vi "VI_Heat_Tape.vi"() -> ()   [LabVIEW 2019]
uses:
  <vilib>/NI/Modbus Library/API/Wrapper/Create Serial Master.vi
  <vilib>/NI/Modbus Library/API/Master/Modbus Master.lvclass
  <vilib>/NI/Modbus Library/API/Wrapper/API Main.lvlib
  <vilib>/NI/Modbus Library/Transmission Data Unit/RTU/RTU Data Unit.lvclass
panel:
  out "Alarm Status":bool
  out "Waveform Chart":dbl(graph)
  out "PXF4 Status":bool
  out "Heater Status":bool
  in  "Upper Threshold (ºF)":string
  in  "Lower Threshold (ºF)":string
  out "Current Temperature Status":bool
  in  "?":bool
  out "Current Temperature (ºF)":string
  out "Heat Tape Temperature (ºF)":dbl(slide) scale=70.0..80.0
  out "Value":sgl
  out "Response Message":string
  out "data string":string
  out "Query Message":string
  in  "unit ID":u8=1
  out "Register and RAW value":u16[](array[numeric])
  in  "number of inputs":u16
  in  "starting address":u16
  in  "error in":errorcluster
  in  "Flow Control":u16(ring) items=["None", "XON/XOFF", "RTS/CTS", "XON/XOFF & RTS/CTS", "DTR/DSR", "XON/XOFF & DTR/DSR"]
  in  "Serial Type":enum16{"RTU", "ASCII"}(ring)
  in  "Parity":u16(ring)=2 items=["None", "Odd", "Even", "Mark", "Space"]
  in  "Baud Rate":u32=9600
  in  "COM Port":refnum<visa-resource-name>
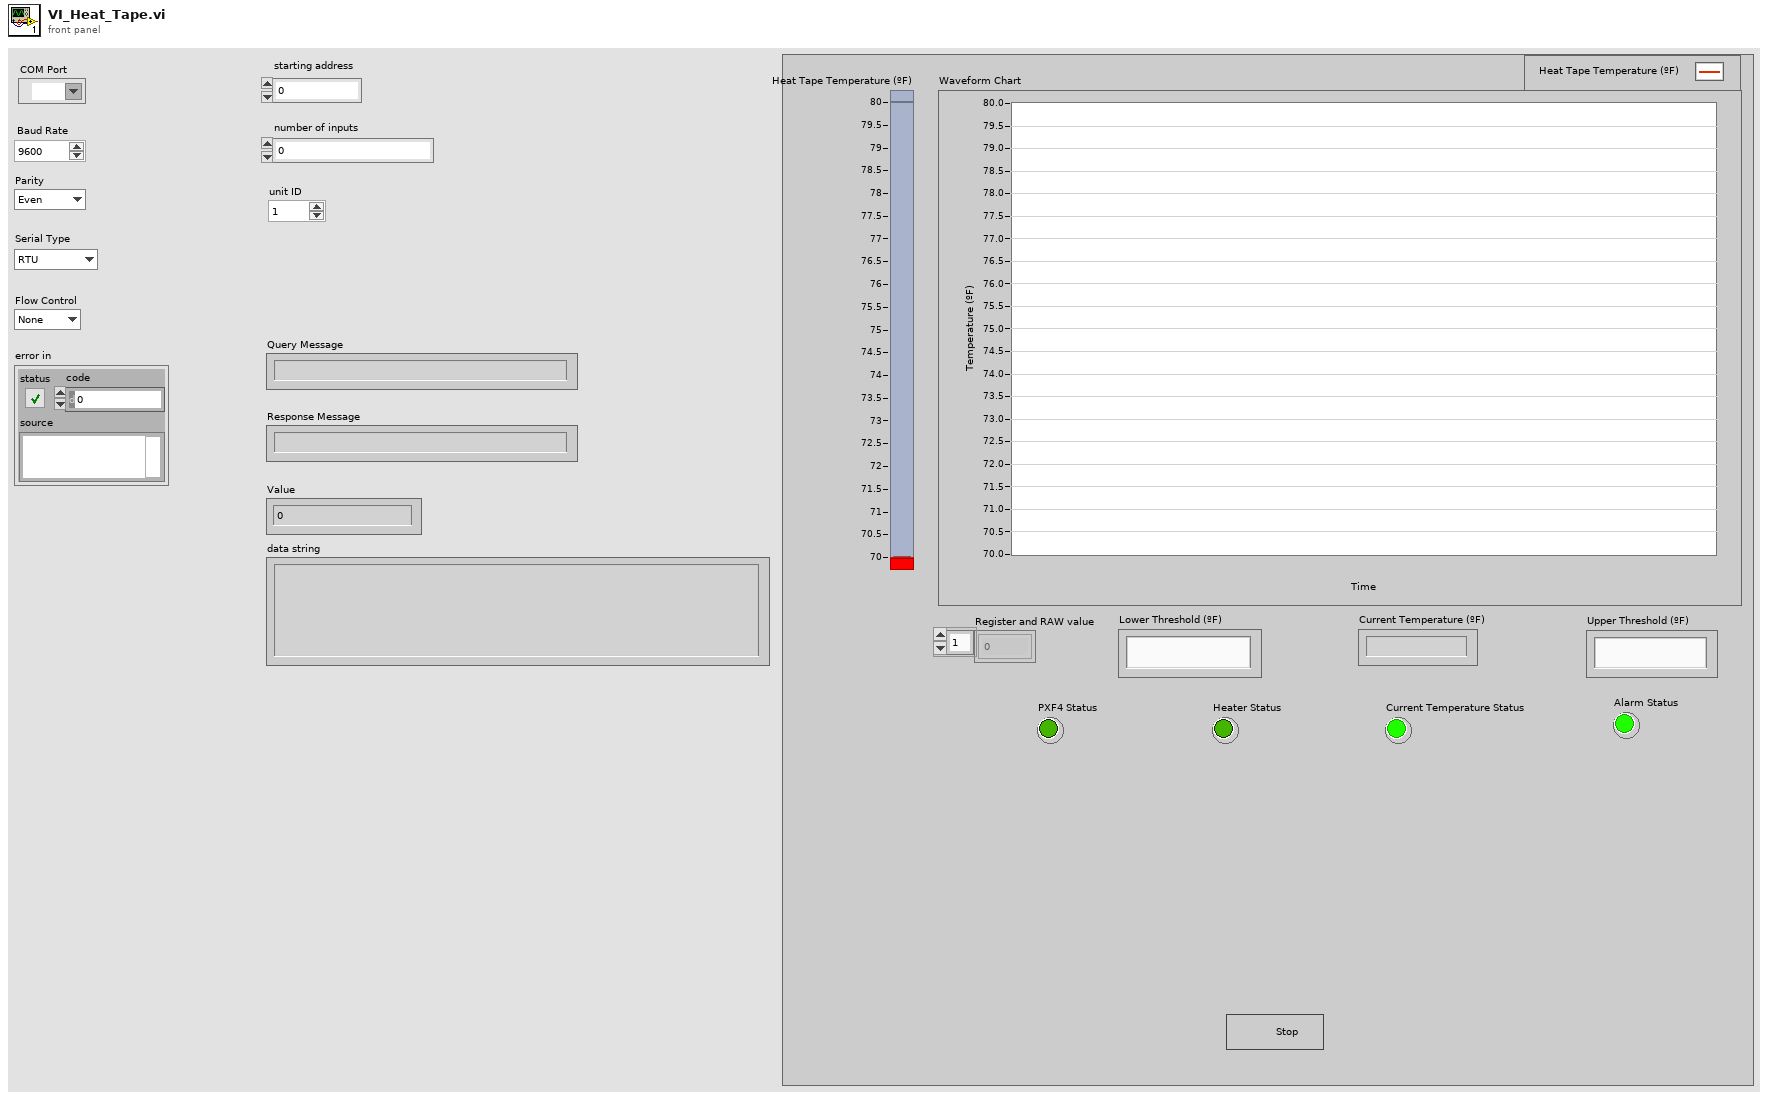
[diagram p1: front panel]
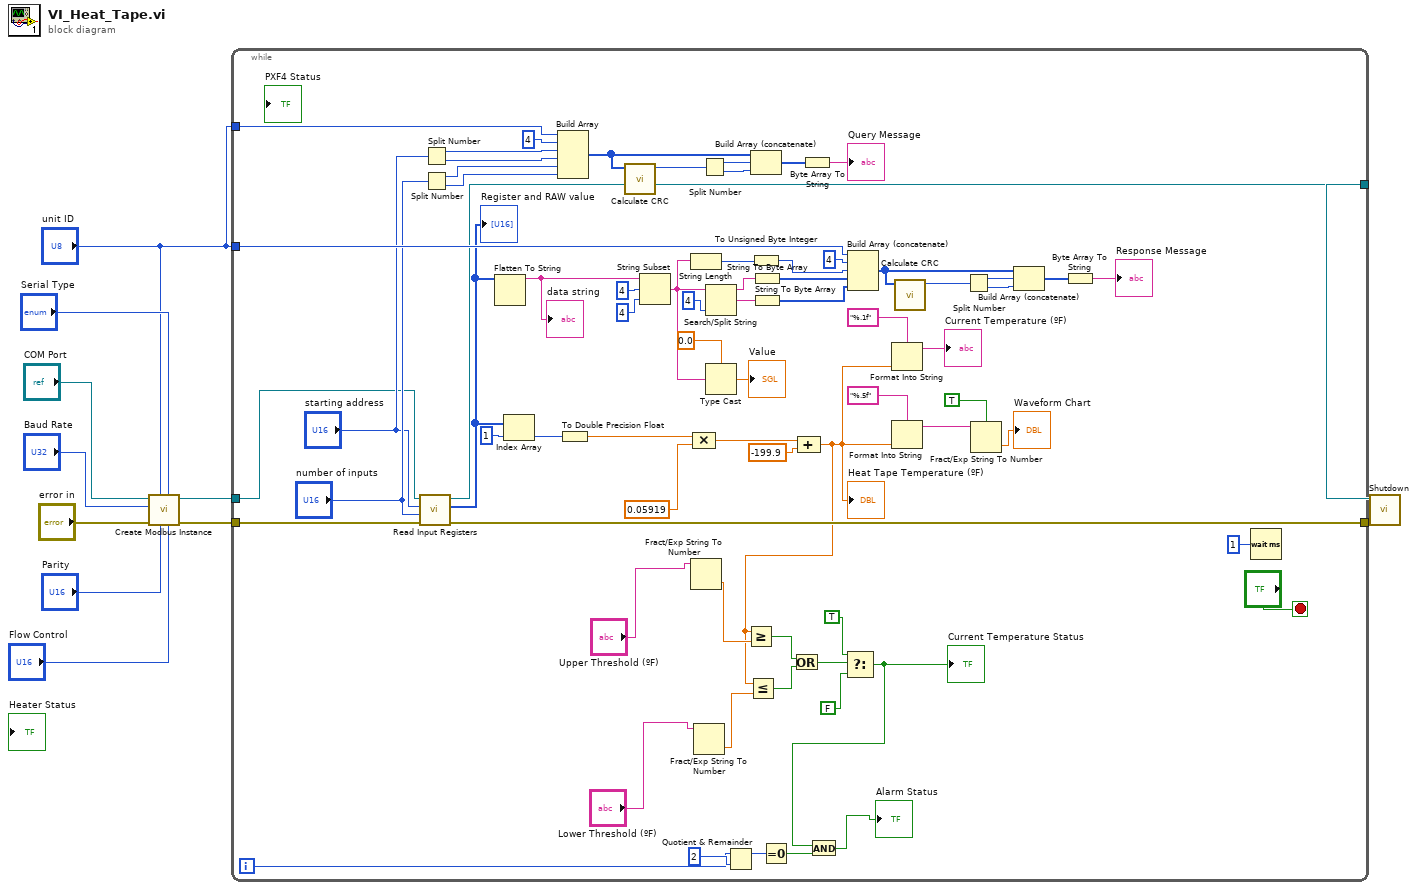
[diagram p0: block diagram]
diagram:
  n1 = call-poly <vilib>:"Create Modbus Instance.vi"("flow control (none)"="Flow Control", "serial type"="Serial Type", "parity (even)"="Parity", "unit ID"="unit ID", "error in"="error in", "baud rate"="Baud Rate", "VISA resource name"="COM Port") -> ("error out"=w5:errorcluster, "serial master instance"=w6:refnum<class "Modbus Master.lvclass">)  [unwired: 3 in]
  n2 = while {
    tunnel: w6 -> [w42]
    tunnel: w5 -> [w47]
    tunnel: [w46] -> w3
    tunnel: [w45] -> w2
    tunnel: "unit ID" -> [w81]
    tunnel: "unit ID" -> [w65]
    i -> [w15]
    stop <- "?" stop-if-true
    n3 = call-dynamic "Read Input Registers.vi"("error in"=w47, "number of inputs"="number of inputs", "starting address"="starting address", "Modbus master in"=w42) -> ("error out"=w46:errorcluster, "register values"=w40:u16[], "Modbus master out"=w45:refnum<class "Modbus Master.lvclass">)  [unwired: 5 in]
    "Register and RAW value" <- w40
    n4 = Split Number(x="starting address") -> (hi(x)=w73:u8, lo(x)=w72:u8)
    n5 = Split Number(x="number of inputs") -> (hi(x)=w71:u8, lo(x)=w70:u8)
    n6 = Flatten To String(anything=w40) -> (data string=w68:string)  [unwired: 3 in, 2 out]
    "data string" <- w68
    n7 = Index Array(array=w40, index=1) -> (element=w36:u16)
    n8 = Build Array(w81, u8 4 ("element"), w73, w72, w71, w70) -> (w79:u8[])
    n9 = To Double Precision Float(number=w36) -> (double precision float=w34:dbl)
    n10 = call <vilib>:"Calculate CRC.vi"("data"=w79) -> ("CRC-16"=w78:u16)  [unwired: 10 in]
    n11 = String Subset(string=w68, offset (0)=4, length (rest)=4 ("length (rest)")) -> (substring=w52:string)
    n12 = String Length(string=w52) -> (length=w66:i32)
    n13 = Fract/Exp String To Number(string="Upper Threshold (ºF)") -> (number=w19:dbl)  [unwired: 3 in, 1 out]
    n14 = Compound Arithmetic op=MULTIPLY(w34, 0.05919 ("value")) -> (w38:dbl)
    n15 = Fract/Exp String To Number(string="Lower Threshold (ºF)") -> (number=w25:dbl)  [unwired: 3 in, 1 out]
    n16 = Split Number(x=w78) -> (hi(x)=w77:u8, lo(x)=w76:u8)
    n17 = Search/Split String(string=w52, offset (0)=4) -> (substring before match=w62:string, match + rest of string=w61:string)  [unwired: 1 in, 1 out]
    n18 = Type Cast(type=sgl 0.0, x=w52) -> (*(type *) &x=→"Value":sgl)
    n19 = Quotient & Remainder(x=w15, y=2) -> (x-y*floor(x/y)=w17:i32)  [unwired: 1 out]
    n20 = Build Array (concatenate)(w79, w77, w76) -> (w75:u8[])
    n21 = To Unsigned Byte Integer(number=w66) -> (unsigned 8bit integer=w63:u8)
    n22 = String To Byte Array(string=w62) -> (unsigned byte array=w60:u8[])
    n23 = String To Byte Array(string=w61) -> (unsigned byte array=w59:u8[])
    n24 = Equal To 0?(x=w17) -> (x = 0?=w14:bool)
    n25 = Compound Arithmetic op=ADD(w38, -199.9 ("value")) -> (w18:dbl)
    "Heat Tape Temperature (ºF)" <- w18
    n26 = Greater Or Equal?(x=w18, y=w19) -> (x >= y?=w24:bool)
    n27 = Less Or Equal?(x=w18, y=w25) -> (x <= y?=w23:bool)
    n28 = Or(x=w24, y=w23) -> (x .or. y?=w22:bool)
    n29 = Byte Array To String(unsigned byte array=w75) -> (string=→"Query Message":string)
    n30 = Select(t=TRUE, s=w22, f=FALSE) -> (s? t:f=w13:bool)
    "Current Temperature Status" <- w13
    n31 = And(x=w13, y=w14) -> (x .and. y?=→"Alarm Status":bool)
    n32 = Build Array (concatenate)(w65, u8 4 ("element"), w63, w60, w59) -> (w53:u8[])
    n33 = Format Into String(format string="%.1f", w18) -> (resulting string=→"Current Temperature (ºF)":string)  [unwired: 2 in, 1 out]
    n34 = Format Into String(format string="%.5f", w18) -> (resulting string=w29:string)  [unwired: 2 in, 1 out]
    n35 = call <vilib>:"Calculate CRC.vi"("data"=w53) -> ("CRC-16"=w54:u16)  [unwired: 10 in]
    n36 = Split Number(x=w54) -> (hi(x)=w55:u8, lo(x)=w56:u8)
    n37 = Fract/Exp String To Number(use system decimal point (T)=TRUE, string=w29) -> (number=→"Waveform Chart":dbl)  [unwired: 2 in, 1 out]
    n38 = Build Array (concatenate)(w53, w55, w56) -> (w57:u8[])
    n39 = Byte Array To String(unsigned byte array=w57) -> (string=→"Response Message":string)
    n40 = Wait (ms)(milliseconds to wait=u32 1) -> ()  [unwired: 1 out]
  }
  n41 = call-dynamic "Shutdown.vi"("error in"=w3, "Modbus master in"=w2) -> ()  [unwired: 9 in, 1 out]
